vi "Test TCP Server.vi"() -> ()   [LabVIEW 2015]
panel:
  out "remote address":string
  out "remote port":u16
  out "Formated shot data":string
  in  "Stop TCP server":bool
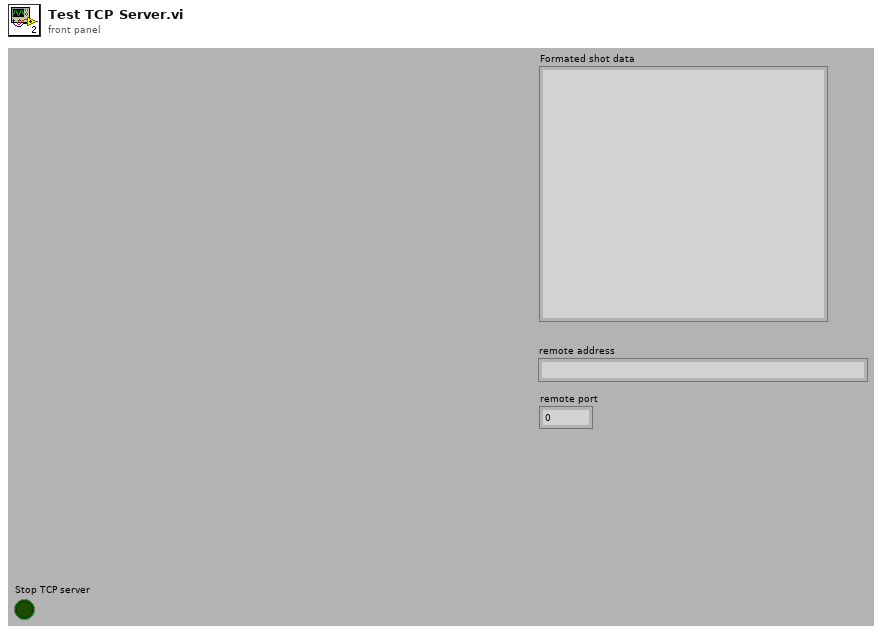
[diagram p1: front panel]
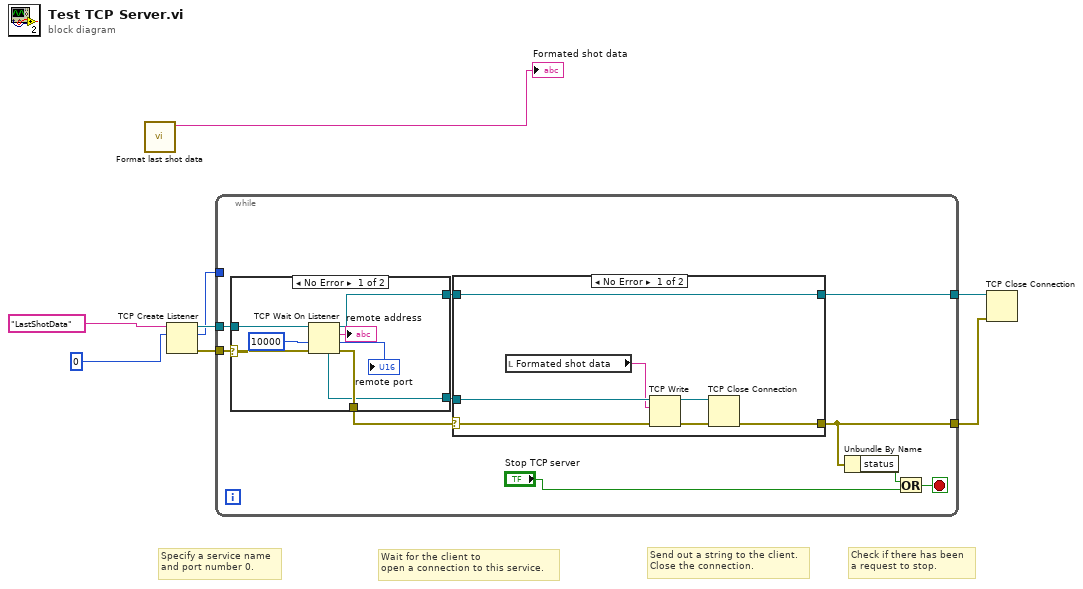
[diagram p0: block diagram]
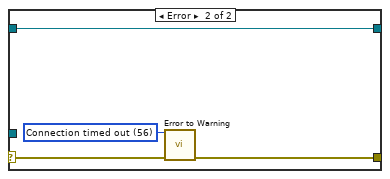
[diagram p2: hidden frame]
diagram:
  # "Check if there has been\na request to stop."
  # "Wait for the client to\nopen a connection to this service."
  # "Send out a string to the client.\nClose the connection."
  # "Specify a service name\nand port number 0."
  n1 = call "Format last shot data.vi"() -> ("Formated shot data"=→"Formated shot data":string)  [unwired: 7 in, 4 out]
  n2 = TCP Create Listener(10:u16 0, 11:"LastShotData") -> (0:w5:errorcluster, 2:w4:u16, 3:w6:refnum<k5>)  [unwired: 3 in]
  n3 = while {
    tunnel: w6 -> [w18]
    tunnel: w5 -> [w16]
    tunnel: [w10] -> w2
    tunnel: w4 -> [_]
    tunnel: [w14] -> w3
    stop <- w12 stop-if-true
    n4 = case shown="No Error" w16 {
      selector: w16 -> [w36 w38]
      tunnel: w18 -> [w37 _]
      tunnel: [w35 w38] -> w13
      tunnel: [w34 _] -> w17
      tunnel: [w32 _] -> w15
      frame No Error {
        n5 = TCP Wait On Listener(8:w36, 9:10000, 11:w37) -> (0:w35:errorcluster, 1:→"remote port":u16, 2:→"remote address":string, 3:w32:refnum<k5>, 4:w34:refnum<k5>)  [unwired: 1 in]
      }
      frame Error {
      }
    }
    n6 = case shown="No Error" w13 {
      selector: w13 -> [w21 w27]
      tunnel: [w24 w26] -> w10
      tunnel: w17 -> [w25 _]
      tunnel: [w20 w29] -> w14
      tunnel: w15 -> [w20 w29]
      frame No Error {
        n7 = local read "Formated shot data"() -> (w19:string)
        n8 = TCP Write(connection ID=w25, data in=w19, error in (no error)=w21) -> (connection ID out=w22:refnum<k5>, error out=w23:errorcluster)  [unwired: 1 in, 1 out]
        n9 = TCP Close Connection(connection ID=w22, error in (no error)=w23) -> (error out=w24:errorcluster)  [unwired: 1 in, 1 out]
      }
      frame Error {
        w28 = 56 items=["No Error", "Argument Error", "Memory Full", "Out of Zone", "End of File", "File Already Open", "Generic File IO Error", "File Not Found", "File Permission Error", "Disk Full", "Duplicate Path", "Too Many Files Open", "Not Enabled", "Resource File Not Found", "Cannot Add Resource", "Resource Not Found", "Image Not Found", "Image Memory Error", "Pen Does Not Exist", "Config Bad Type", "Config Token Not Found", "Config Parse Error", "Config Memory Error", "Bad External Code Format", "Bad External Code Offset", "External Code Not Present", "Null Window", "Destroy Window Mixup", "Null Menu", "Print Aborted", "Bad Print Record", "Print Driver Error", "Windows Error During Print", "Memory Error During Print", "Print Dialog Error", "Generic Print Error", "Invalid Device Refnum", "Device Not Found", "Device Parameter Error", "Device Unit Error", "Can't Open Device", "Device Call Aborted", "Generic Error", "Cancelled By User", "Object ID Too Low", "Object ID Too High", "Object Not In Heap", "Unknown Heap", "Bad DefProc ID", "DefProc Not In Table", "Message Out Of Range", "Null Method", "Unknown Message", "Manager Call Not Supported", "Bad address", "Connection In progress", "Connection timed out", "Connection is already in progress", "Network attribute not supported", "Network error", "Address in use", "System out of memory", "Connection aborted", "Connection refused", "Connection is not connected", "Connection is already connected", "Connection closed", "Initialize error (interapplication manager)", "Bad occurrence", "Wait on unbound occurrence handler", "Occurrence queue overflow", "Bad path", "Semaphore not signaled", "Unrecognized type (interapplication manager)"] ("1st Error to Convert")
        n10 = call <vilib>:"Error to Warning.vi"("1st Error to Convert"=w28, "error in"=w27) -> ("warning out"=w26:errorcluster)  [unwired: 13 in]
      }
    }
    n11 = Unbundle By Name(w10) -> ("status"=w11:bool)
    n12 = Or(x=w11, y="Stop TCP server") -> (x .or. y?=w12:bool)
  }
  n13 = TCP Close Connection(connection ID=w3, error in (no error)=w2) -> ()  [unwired: 1 in, 2 out]
